vi "DTCs.Codes.Get.vi"(8 "error in (no error)":errorcluster, 10 "Addon Name":string, 11 "Address":string) -> (0 "error out":errorcluster, 3 "Codes":T1)   [LabVIEW 2019, in "Diagnostics Addon Shared.lvlib"]
uses:
  Diagnostics Addon Shared.lvlib
  Types/DTC.Codes.ctl
  NationalInstruments.VeriStand.SystemDefinitionAPI
  NationalInstruments.VeriStand.SystemStorage
  Constants.vi
  <vilib>/NI VeriStand/Execution/Workspace/NI_VS Workspace ExecutionAPI.lvlib
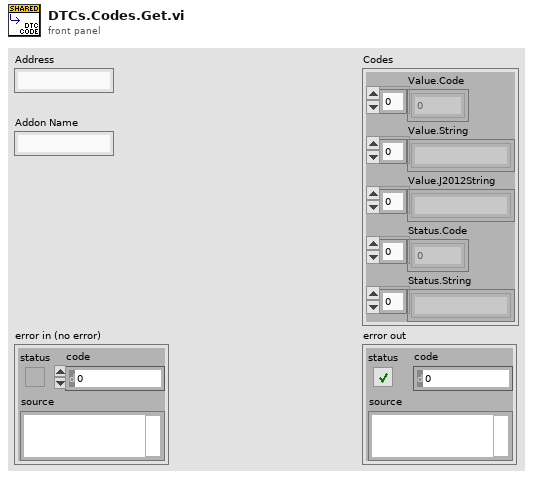
[diagram p1: front panel]
types:
  T1 = typedef "Diagnostics Addon Shared.lvlib/DTC.Codes.ctl" = cluster{"Value.Code":dbl[], "Value.String":string[], "Value.J2012String":string[], "Status.Code":dbl[], "Status.String":string[]}
  T2 = typedef "NI_VS Workspace ExecutionAPI.lvlib/WorkspaceAPI.ctl" = refnum<k24>
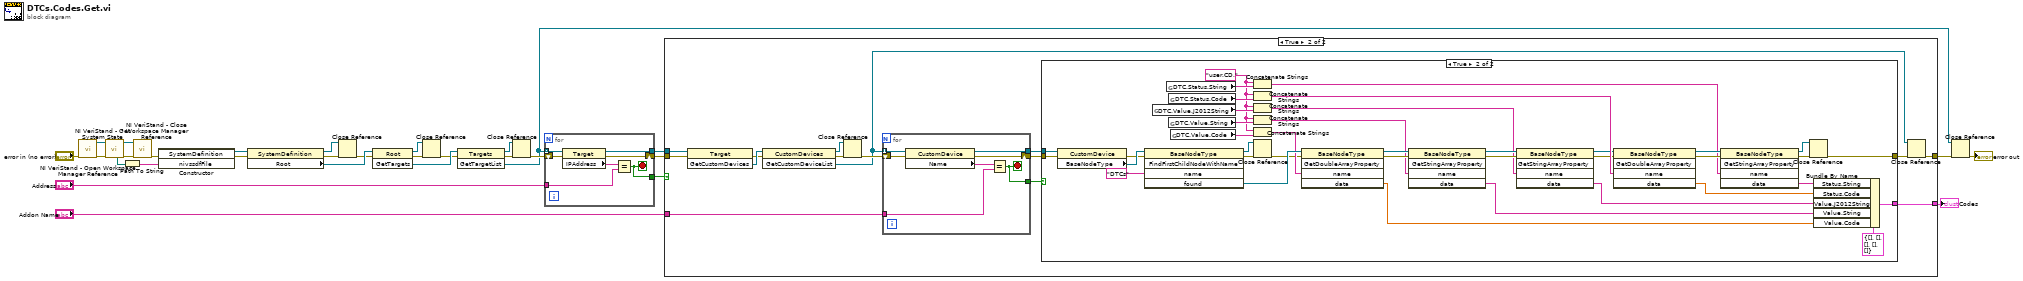
[diagram p0: block diagram]
diagram:
  n1 = call <vilib>:"NI VeriStand - Open Workspace Manager Reference.vi"("error in (no error)"="error in (no error)") -> ("error out"=w30:errorcluster, "WorkspaceManager"=w29:T2)  [unwired: 9 in]
  n2 = call <vilib>:"NI VeriStand - Get System State.vi"("error in (no error)"=w30, "WorkspaceManager in"=w29) -> ("error out"=w28:errorcluster, "WorkspaceManager  out"=w27:T2, "System Definition File"=w26:path)  [unwired: 5 in, 2 out]
  n3 = Path To String(path=w26) -> (string=w25:string)
  n4 = call <vilib>:"NI VeriStand - Close Workspace Manager Reference.vi"("error in (no error)"=w28, "WorkspaceManager"=w27) -> ("error out"=w24:errorcluster)  [unwired: 9 in]
  n5 = constructor class="SystemDefinition"(error in=w24, "nivssdfFile"=w25) -> (reference out=w23:refnum<k24>, error out=w22:errorcluster)  [unwired: 2 in, 2 out]
  n6 = property class="SystemDefinition"(reference=w23, error in=w22) -> (reference out=w17:refnum<k24>, error out=w16:errorcluster, "Root"=w21:refnum<k24>)
  n7 = Close Reference(reference=w17, error in (no error)=w16) -> (error out=w15:errorcluster)
  n8 = invoke class="Root" method="GetTargets"(reference=w21, error in=w15) -> (reference out=w12:refnum<k24>, error out=w14:errorcluster, "GetTargets"=w20:refnum<k24>)  [unwired: 1 in]
  n9 = Close Reference(reference=w12, error in (no error)=w14) -> (error out=w13:errorcluster)
  n10 = invoke class="Targets" method="GetTargetList"(reference=w20, error in=w13) -> (reference out=w9:refnum<k24>, error out=w11:errorcluster, "GetTargetList"=w6:refnum<k24>[])  [unwired: 1 in]
  n11 = Close Reference(reference=w9, error in (no error)=w11) -> (error out=w10:errorcluster)
  n12 = for {
    tunnel: w6 -> [w37] mode=indexing
    shift-right: [w35] -> w8
    shift-left: w10 -> [w36]
    tunnel: "Address" -> [w33]
    tunnel: [w32] -> w19
    tunnel: [w31] -> w18
    stop <- w32 stop-if-true
    n13 = property class="Target"(reference=w37, error in=w36) -> (reference out=w31:refnum<k24>, error out=w35:errorcluster, "IPAddress"=w34:string)
    n14 = Equal?(x=w34, y=w33) -> (x = y?=w32:bool)
  }
  n15 = case shown="True" w19 {
    tunnel: w18 -> [_ w53]
    tunnel: w8 -> [w38 w52]
    tunnel: "Addon Name" -> [_ w49]
    tunnel: [w38 w40] -> w7
    tunnel: [_ w39] -> w4
    frame False {
    }
    frame True {
      n16 = invoke class="Target" method="GetCustomDevices"(reference=w53, error in=w52) -> (error out=w50:errorcluster, "GetCustomDevices"=w51:refnum<k24>)  [unwired: 1 in, 1 out]
      n17 = invoke class="CustomDevices" method="GetCustomDeviceList"(reference=w51, error in=w50) -> (reference out=w43:refnum<k24>, error out=w45:errorcluster, "GetCustomDeviceList"=w41:refnum<k24>[])  [unwired: 1 in]
      n18 = Close Reference(reference=w43, error in (no error)=w45) -> (error out=w44:errorcluster)
      n19 = for {
        tunnel: w41 -> [w99] mode=indexing
        shift-right: [w97] -> w46
        shift-left: w44 -> [w98]
        tunnel: w49 -> [w95]
        tunnel: [w94] -> w48
        tunnel: [w93] -> w47
        stop <- w94 stop-if-true
        n20 = property class="CustomDevice"(reference=w99, error in=w98) -> (reference out=w93:refnum<k24>, error out=w97:errorcluster, "Name"=w96:string)
        n21 = Equal?(x=w96, y=w95) -> (x = y?=w94:bool)
      }
      n22 = case shown="True" w48 {
        tunnel: w47 -> [_ w92]
        tunnel: w46 -> [w54 w91]
        tunnel: [w54 w69] -> w42
        tunnel: [_ w63] -> w39
        frame False {
        }
        frame True {
          w57 = "user.CD."
          n23 = property class="CustomDevice"(reference=w92, error in=w91) -> (error out=w89:errorcluster, "BaseNodeType"=w90:refnum<k24>)  [unwired: 1 out]
          n24 = invoke class="BaseNodeType" method="FindFirstChildNodeWithName"(reference=w90, error in=w89, "name"="DTCs") -> (reference out=w74:refnum<k24>, error out=w73:errorcluster, "found"=w87:refnum<k24>)  [unwired: 2 in, 2 out]
          n25 = global read "Constants.vi" "DTC.Value.J2012String"() -> (w58:string)
          n26 = global read "Constants.vi" "DTC.Status.String"() -> (w79:string)
          n27 = global read "Constants.vi" "DTC.Status.Code"() -> (w80:string)
          n28 = global read "Constants.vi" "DTC.Value.String"() -> (w81:string)
          n29 = global read "Constants.vi" "DTC.Value.Code"() -> (w82:string)
          n30 = Concatenate Strings(w57, w79) -> (w75:string)
          n31 = Concatenate Strings(w57, w80) -> (w76:string)
          n32 = Concatenate Strings(w57, w58) -> (w56:string)
          n33 = Concatenate Strings(w57, w81) -> (w77:string)
          n34 = Concatenate Strings(w57, w82) -> (w78:string)
          n35 = Close Reference(reference=w74, error in (no error)=w73) -> (error out=w72:errorcluster)
          n36 = invoke class="BaseNodeType" method="GetDoubleArrayProperty"(reference=w87, error in=w72, "name"=w78) -> (reference out=w85:refnum<k24>, error out=w86:errorcluster, "data"=w67:dbl[])  [unwired: 2 in, 2 out]
          n37 = invoke class="BaseNodeType" method="GetStringArrayProperty"(reference=w85, error in=w86, "name"=w77) -> (reference out=w61:refnum<k24>, error out=w62:errorcluster, "data"=w66:string[])  [unwired: 2 in, 2 out]
          n38 = invoke class="BaseNodeType" method="GetStringArrayProperty"(reference=w61, error in=w62, "name"=w56) -> (reference out=w60:refnum<k24>, error out=w59:errorcluster, "data"=w55:string[])  [unwired: 2 in, 2 out]
          n39 = invoke class="BaseNodeType" method="GetDoubleArrayProperty"(reference=w60, error in=w59, "name"=w76) -> (reference out=w84:refnum<k24>, error out=w83:errorcluster, "data"=w65:dbl[])  [unwired: 2 in, 2 out]
          n40 = invoke class="BaseNodeType" method="GetStringArrayProperty"(reference=w84, error in=w83, "name"=w75) -> (reference out=w70:refnum<k24>, error out=w71:errorcluster, "data"=w64:string[])  [unwired: 2 in, 2 out]
          n41 = Close Reference(reference=w70, error in (no error)=w71) -> (error out=w69:errorcluster)
          n42 = Bundle By Name(cluster=T1 {"Value.Code"=[], "Value.String"=[], "Value.J2012String"=[], "Status.Code"=[], "Status.String"=[]}, "Status.String"=w64, "Status.Code"=w65, "Value.J2012String"=w55, "Value.String"=w66, "Value.Code"=w67) -> (w63:T1)
        }
      }
      n43 = Close Reference(reference=w41, error in (no error)=w42) -> (error out=w40:errorcluster)
    }
  }
  "Codes" <- w4
  n44 = Close Reference(reference=w6, error in (no error)=w7) -> (error out=→"error out":errorcluster)
